vi "solar_qtimer Find.vi"(10 "QTimer":string, 11 "QTimer Settings":T1[](array[typedef])) -> (2 "Exists?":bool, 3 "Index":i32)   [LabVIEW 2018]
doc: "This searches for a QTimer by name."
uses:
  solar_qtimer_ctl QTimer Settings.ctl
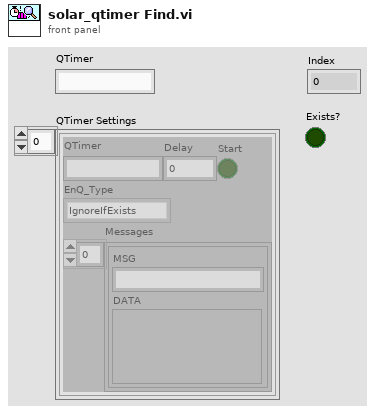
[diagram p1: front panel]
types:
  T1 = typedef "solar_qtimer_ctl QTimer Settings.ctl" = cluster{"QTimer":string, "Delay":i32, "Start":bool, "EnQ_Type":enum8{"Normal", "Priority", "IgnoreIfExists"}, "Messages":cluster{"MSG":string, "DATA":variant}[]}
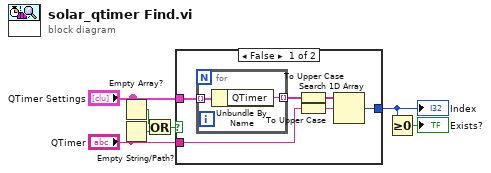
[diagram p0: block diagram]
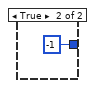
[diagram p2: hidden frame]
diagram:
  n1 = Empty Array?(array="QTimer Settings") -> (empty?=w4:bool)
  n2 = Empty String/Path?(string/path="QTimer") -> (empty?=w1:bool)
  n3 = Or(x=w4, y=w1) -> (x .or. y?=w2:bool)
  n4 = case shown="False" w2 {
    tunnel: "QTimer Settings" -> [w13 _]
    tunnel: "QTimer" -> [w9 _]
    tunnel: [w8 -1 ("index of element")] -> w7
    frame False {
      n5 = for {
        tunnel: w13 -> [w15] mode=indexing
        tunnel: [w14] -> w12 mode=indexing
        n6 = Unbundle By Name(w15) -> ("QTimer"=w14:string)
      }
      n7 = To Upper Case(1:w12) -> (0:w11:string[])
      n8 = To Upper Case(1:w9) -> (0:w10:string)
      n9 = Search 1D Array(1D array=w11, element=w10) -> (index of element=w8:i32)  [unwired: 1 in]
    }
    frame True {
    }
  }
  "Index" <- w7
  n10 = Greater Or Equal To 0?(x=w7) -> (x >= 0?=→"Exists?":bool)
